vi "Parameter Estimation.vi"() -> ()   [LabVIEW 2009]
panel:
  out "A":dbl[](array[numeric])
  out "C":dbl[](array[numeric])
  out "B":dbl[](array[numeric])
  out "Numeric":i32
  out "E(k)":dbl
  in  "stop":bool
  in  "Learn Rate":dbl=0.1
  out "M(k)":dbl
  out "M^(k)":dbl
  in  "Order":i32=3
  in  "Empty Dryer Cold Weight":dbl
  in  "Bone Dry Weight":dbl
  in  "Weigth":string
  in  "T RDB":string
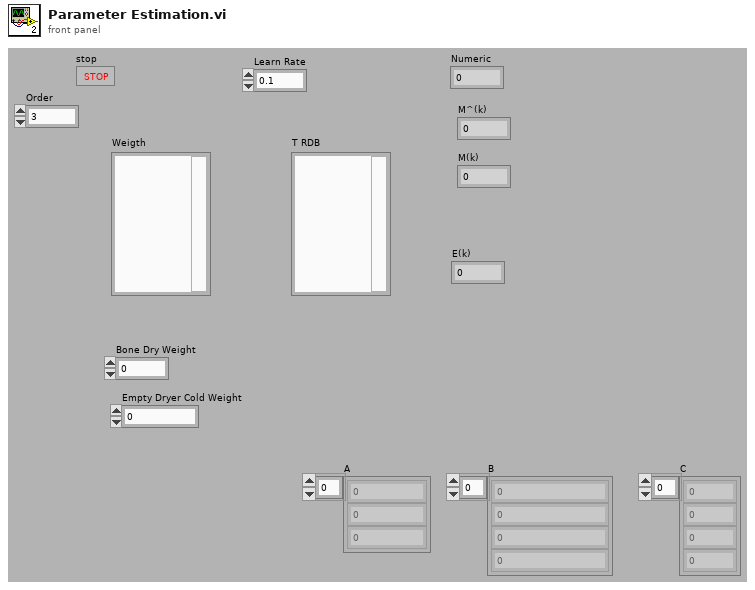
[diagram p1: front panel]
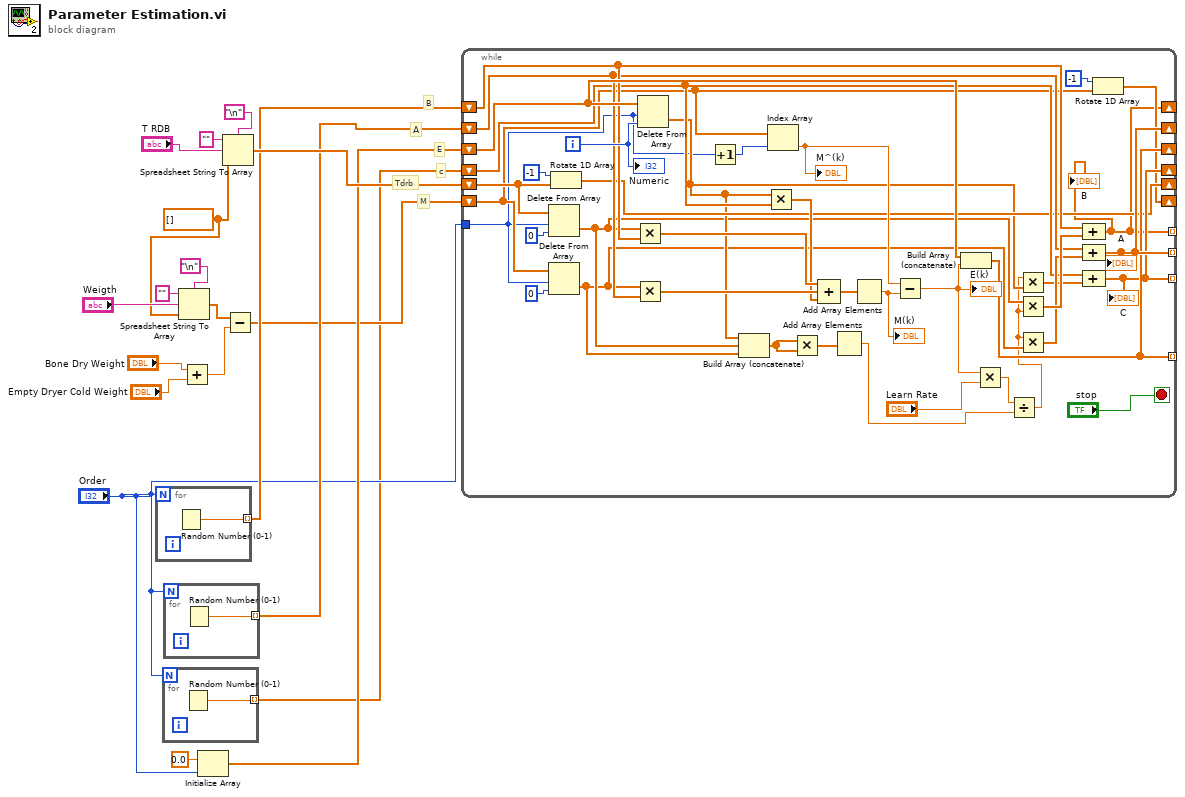
[diagram p0: block diagram]
diagram:
  w12 = dbl[] [] ("array type (2D Dbl)")
  # "c"
  # "E"
  # "A"
  # "M"
  # "Tdrb"
  # "B"
  n1 = for {
    N: "Order" -> [_]
    tunnel: [w20] -> w11 mode=indexing
    n2 = Random Number (0-1)() -> (number: 0 to 1=w20:dbl)
  }
  n3 = for {
    N: "Order" -> [_]
    tunnel: [w21] -> w1 mode=indexing
    n4 = Random Number (0-1)() -> (number: 0 to 1=w21:dbl)
  }
  n5 = for {
    N: "Order" -> [_]
    tunnel: [w22] -> w10 mode=indexing
    n6 = Random Number (0-1)() -> (number: 0 to 1=w22:dbl)
  }
  n7 = Spreadsheet String To Array(delimiter (Tab)="\n", format string="", spreadsheet string="Weigth", array type (2D Dbl)=w12) -> (array=w6:dbl[])
  n8 = Add(x="Bone Dry Weight", y="Empty Dryer Cold Weight") -> (x+y=w5:dbl)
  n9 = Initialize Array(0.0 ("element"), "Order") -> (w9:dbl[])
  n10 = Spreadsheet String To Array(delimiter (Tab)="\n", format string="", spreadsheet string="T RDB", array type (2D Dbl)=w12) -> (array=w13:dbl[])
  n11 = Subtract(x=w6, y=w5) -> (x-y=w4:dbl[])
  n12 = while {
    tunnel: "Order" -> [w23]
    shift-right: [w25] -> _
    shift-left: w11 -> [w51]
    shift-right: [w46] -> _
    shift-left: w10 -> [w49]
    shift-right: [w45] -> _
    shift-left: w9 -> [w56]
    shift-right: [w44] -> _
    shift-left: w1 -> [w48]
    tunnel: [w25] -> _ mode=indexing
    tunnel: [w46] -> _ mode=indexing
    tunnel: [w45] -> _ mode=indexing
    tunnel: [w44] -> _ mode=indexing
    shift-right: [w41] -> _
    shift-left: w13 -> [w42]
    shift-right: [w38] -> _
    shift-left: w4 -> [w37]
    i -> [w55]
    stop <- "stop" stop-if-true
    n13 = Delete From Array(array=w42, length=w23, index=0) -> (deleted portion=w33:dbl[])  [unwired: 1 out]
    n14 = Delete From Array(array=w37, length=w23, index=0) -> (deleted portion=w32:dbl[])  [unwired: 1 out]
    n15 = Rotate 1D Array(1:w42, 2:-1 ("n")) -> (0:w41:dbl[])
    n16 = Multiply(x=w33, y=w51) -> (x*y=w61:dbl[])
    n17 = Multiply(x=w32, y=w49) -> (x*y=w60:dbl[])
    n18 = Delete From Array(array=w56, length=w23, index=w55) -> (deleted portion=w34:dbl[])  [unwired: 1 out]
    n19 = Increment(x=w23) -> (x+1=w24:i32)
    n20 = Build Array (concatenate)(w34, w33, w32) -> (w31:dbl[])
    n21 = Multiply(x=w34, y=w48) -> (x*y=w54:dbl[])
    n22 = Index Array(array=w37, index=w24) -> (element=w58:dbl)
    "M^(k)" <- w58
    n23 = Multiply(x=w31, y=w31) -> (x*y=w30:dbl[])
    n24 = Compound Arithmetic op=ADD(w61, w60, w54) -> (w59:dbl[])
    n25 = Add Array Elements(numeric array=w30) -> (sum=w26:dbl)
    n26 = Add Array Elements(numeric array=w59) -> (sum=w57:dbl)
    "M(k)" <- w57
    n27 = Subtract(x=w58, y=w57) -> (x-y=w29:dbl)
    "E(k)" <- w29
    n28 = Build Array (concatenate)(w56, w29) -> (w45:dbl[])
    n29 = Multiply(x=w29, y="Learn Rate") -> (x*y=w27:dbl)
    n30 = Divide(x=w27, y=w26) -> (x/y=w28:dbl)
    n31 = Multiply(x=w28, y=w34) -> (x*y=w47:dbl[])
    n32 = Multiply(x=w33, y=w28) -> (x*y=w52:dbl[])
    n33 = Multiply(x=w28, y=w32) -> (x*y=w50:dbl[])
    n34 = Compound Arithmetic op=ADD(w51, w52) -> (w25:dbl[])
    "B" <- w25
    n35 = Compound Arithmetic op=ADD(w49, w50) -> (w46:dbl[])
    "A" <- w46
    n36 = Compound Arithmetic op=ADD(w48, w47) -> (w44:dbl[])
    "C" <- w44
    n37 = Rotate 1D Array(1:w37, 2:-1 ("n")) -> (0:w38:dbl[])
    "Numeric" <- w55
  }
